vi "test rinse.vi"() -> ()   [LabVIEW 2017]
uses:
  <instrlib>/Harvard Apparatus PHD Ultra Series/Harvard Apparatus PHD Ultra Series.lvlib
  <instrlib>/Harvard Syringe Pump PHD2000/Harvard Syringe Pump PHD2000.lvlib
panel:
  in  "Pump 2 COM":refnum<visa-resource-name>="COM9"
  in  "Pump 1 COM":refnum<visa-resource-name>="COM12"
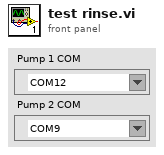
[diagram p1: front panel]
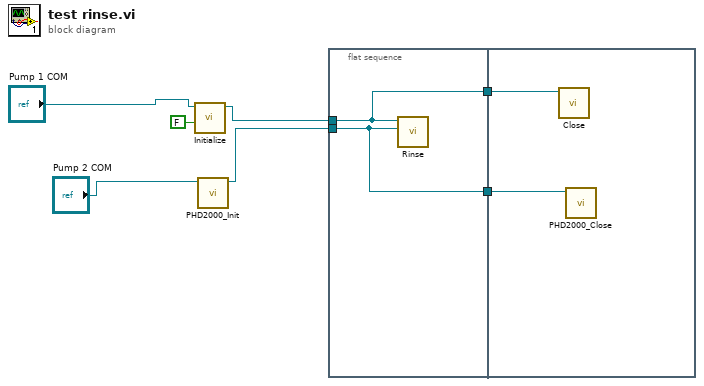
[diagram p0: block diagram]
diagram:
  n1 = call <instrlib>:"Initialize.vi"("ID Query (True)"=FALSE, "VISA resource name"="Pump 1 COM") -> ("VISA resource name out"=w5:refnum<visa-resource-name>)  [unwired: 8 in, 1 out]
  n2 = call <instrlib>:"PHD2000_Init.vi"("VISA resource name"="Pump 2 COM") -> ("reference out"=w3:refnum<visa-resource-name>)  [unwired: 8 in, 1 out]
  n3 = flat-sequence {
    tunnel: w5 -> [w9]
    tunnel: w3 -> [w8]
    tunnel: [w9] -> w2
    tunnel: [w8] -> w1
    tunnel: w2 -> [w11]
    tunnel: w1 -> [w10]
    frame #0 {
      n4 = call "Rinse.vi"("Pump 2 COM"=w8, "Pump 1 COM"=w9) -> ()  [unwired: 10 in]
    }
    frame #1 {
      n5 = call <instrlib>:"Close.vi"("VISA resource name"=w11) -> ()  [unwired: 10 in, 1 out]
      n6 = call <instrlib>:"PHD2000_Close.vi"("VISA resource name"=w10) -> ()  [unwired: 9 in, 1 out]
    }
  }
